vi "CTRE_CANifier_GetLastError.vi"(8 "error in":errorcluster, 11 "CANifierDevRef":T1) -> (0 "error out":errorcluster, 2 "Last Error Code":i8, 3 "CANifierDevRef":T1)   [LabVIEW 2020]
doc: "Returns the last error generated by the CANifier object."
uses:
  <vilib>/Rock Robotics/WPI/ThirdParty/Phoenix-LabVIEW/CANifier/CTRE_CANifier_DeviceRef.ctl
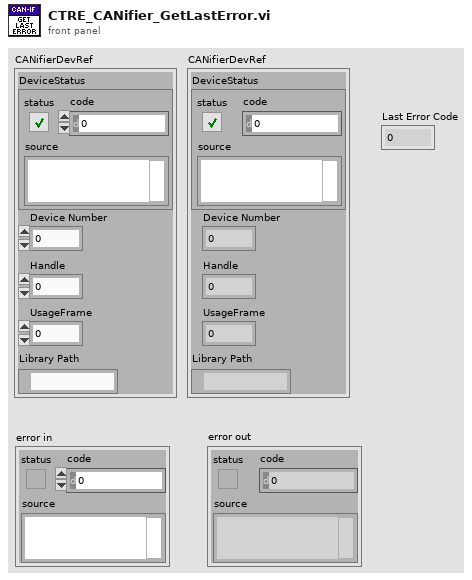
[diagram p1: front panel]
types:
  T1 = typedef "CTRE_CANifier_DeviceRef.ctl" = cluster{"DeviceStatus":errorcluster, "Device Number":u8, "Handle":u64, "UsageFrame":u32, "Library Path":path}
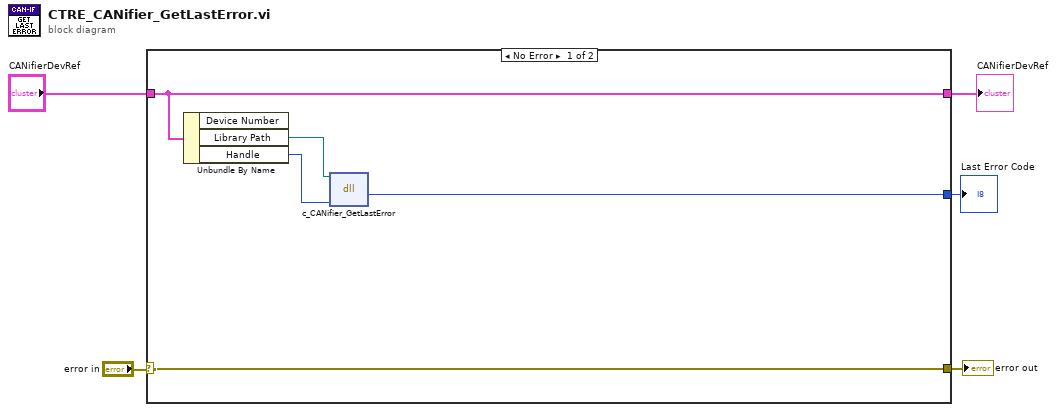
[diagram p0: block diagram]
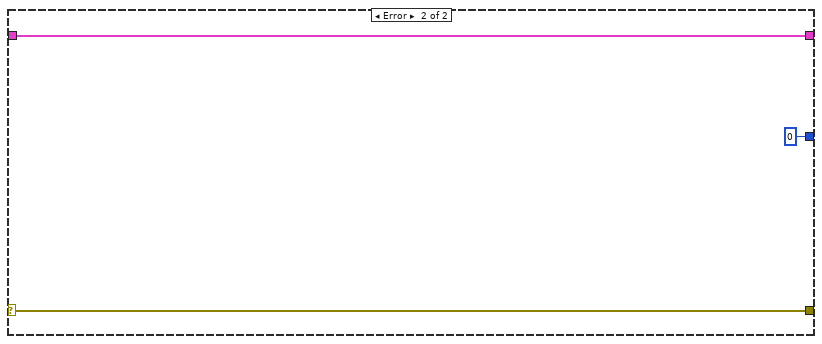
[diagram p2: hidden frame]
diagram:
  n1 = case shown="No Error" "error in" {
    selector: "error in" -> [w10 w13]
    tunnel: [w10 w13] -> w4
    tunnel: "CANifierDevRef" -> [w9 w12]
    tunnel: [w9 w12] -> w2
    tunnel: [w6 i8 0 ("ErrorCode")] -> w1
    frame No Error {
      n2 = Unbundle By Name(w9) -> ("Library Path"=w8:path, "Handle"=w7:u64)  [unwired: 1 out]
      n3 = dll-call lib="?" fn="c_CANifier_GetLastError"(path in=w8, "handle"=w7) -> ("ErrorCode"=w6:i8)  [unwired: 3 in, 2 out]
    }
    frame Error {
    }
  }
  "error out" <- w4
  "CANifierDevRef" <- w2
  "Last Error Code" <- w1
